vi "upateWaitBar.vi"(3 "waitbar text":string, 4 "waitbar value [0,1]":sgl, 5 "Progress":refnum<vi>) -> (2 "Updated Progress":refnum<vi>)   [LabVIEW 2017]
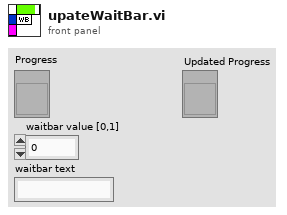
[diagram p1: front panel]
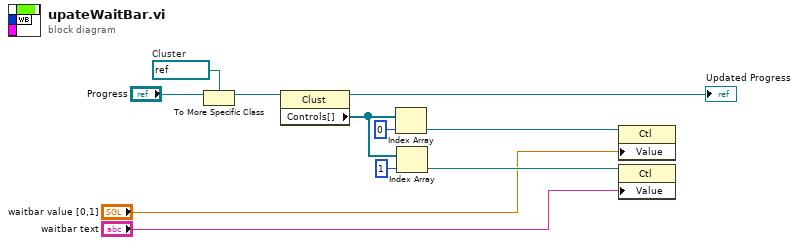
[diagram p0: block diagram]
diagram:
  w11 = refnum<vi> refnum  # Cluster
  n1 = To More Specific Class(target class=w11, reference="Progress") -> (specific class reference=w9:refnum<vi>)  [unwired: 1 in, 1 out]
  n2 = property class="Clust"(reference=w9) -> (reference out=→"Updated Progress":refnum<vi>, "Controls[]"=w6:refnum<vi>[])  [unwired: 1 in, 1 out]
  n3 = Index Array(array=w6, index=0) -> (element=w4:refnum<vi>)
  n4 = Index Array(array=w6, index=1) -> (element=w5:refnum<vi>)
  n5 = property class="Ctl"(reference=w4, "Value"="waitbar value [0,1]") -> ()  [unwired: 1 in, 2 out]
  n6 = property class="Ctl"(reference=w5, "Value"="waitbar text") -> ()  [unwired: 1 in, 2 out]
